vi "Sub_VI_ejecutar_Aula_3.vi"(0 "Serrvicio":u8, 1 "Edif_string_aula":string, 2 "+                 -":bool, 3 "Aula":string, 4 "edo_actual_aula":bool) -> ()   [LabVIEW 2017]
uses:
  GlobalFag.vi
  Global_comSerie.vi
  <vilib>/Instr/_visa.llb/VISA Configure Serial Port (Instr).vi
panel:
  out "aula_ascii":string
  out "estado 3":bool[](array[boolean])
  in  "stop_aula":bool
  in  "Servicios":bool[](array[boolean])
  # "Conf para Edif A, aula 15"
  # "Servicio"
  # "Luz"
  # "+/- Edo. Actual"
  # "Aire"
  # "Proyector"
  # "Agua"
  # "Acceso"
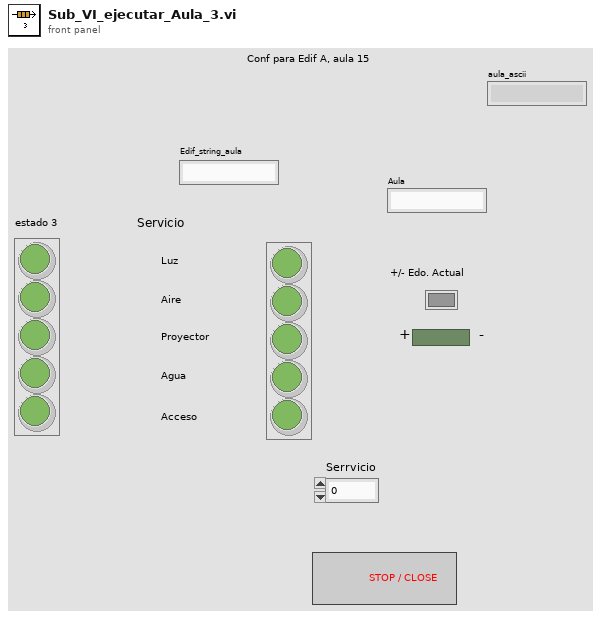
[diagram p1: front panel]
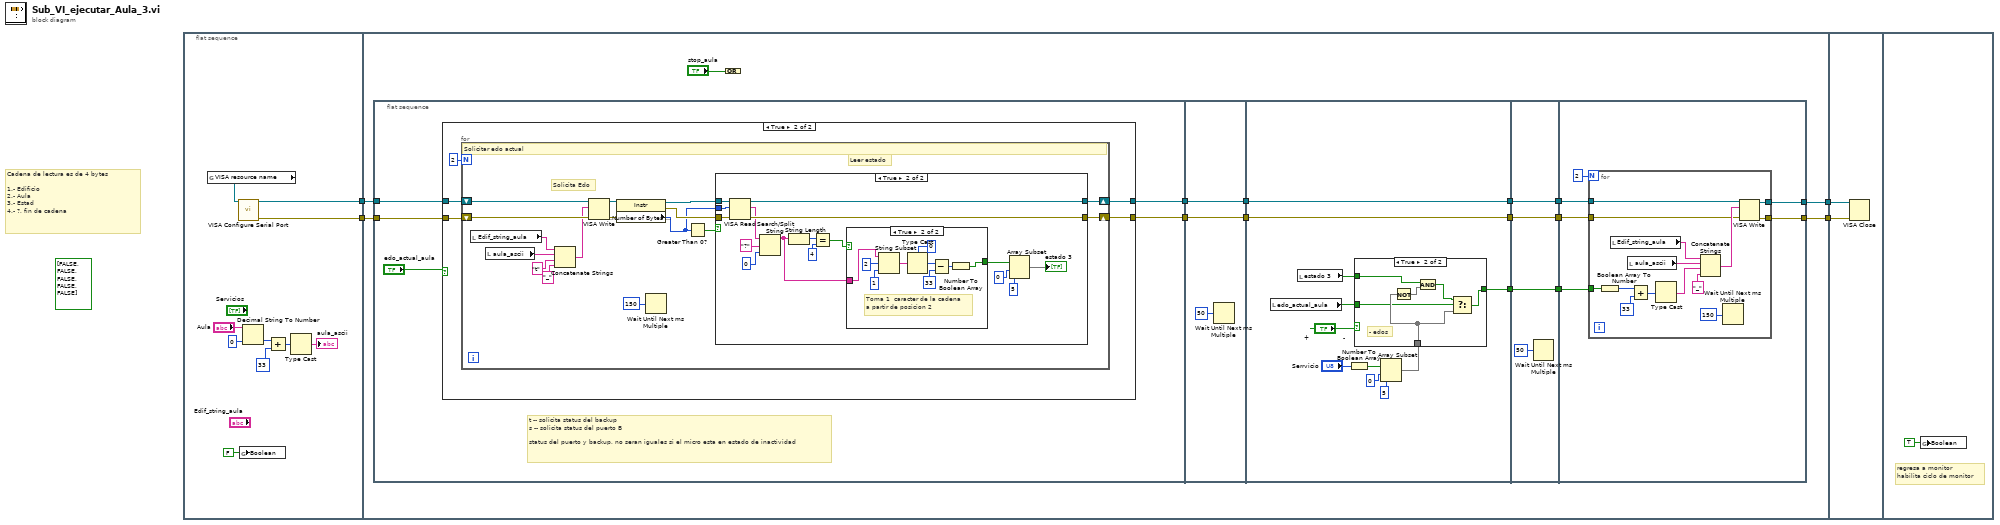
[diagram p0: block diagram]
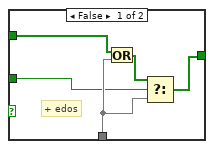
[diagram p5: hidden frame]
diagram:
  (unwired) bool[] [FALSE, FALSE, FALSE, FALSE, FALSE] ("Servicios")
  # "Cadena de lectura es de 4 bytes\n\n1.- Edificio\n2.- Aula\n3.- Estad\n4.- ?, fin de cadena"
  n1 = flat-sequence {
    tunnel: [w14] -> w4
    tunnel: [w13] -> w3
    tunnel: w4 -> [w28]
    tunnel: w3 -> [w27]
    tunnel: [w26] -> w2
    tunnel: [w25] -> w1
    tunnel: w2 -> [w135]
    tunnel: w1 -> [w134]
    frame #0 {
      n2 = global read "Global_comSerie.vi" "VISA resource name"() -> (w11:refnum<visa-resource-name>)
      n3 = call-poly "VISA Configure Serial Port"("VISA resource name"=w11) -> ("VISA resource name out"=w14:refnum<visa-resource-name>, "error out"=w13:errorcluster)  [unwired: 13 in]
      n4 = global write "GlobalFag.vi" "Boolean"(FALSE ("Boolean")) -> ()
      n5 = Decimal String To Number(string="Aula", default (0L)=u8 0 ("default (0 I32)")) -> (number=w8:u8)  [unwired: 1 in, 1 out]
      n6 = Add(x=w8, y=u8 33) -> (x+y=w6:u8)
      n7 = Type Cast(x=w6) -> (*(type *) &x=→"aula_ascii":string)  [unwired: 1 in]
    }
    frame #1 {
      n8 = flat-sequence {
        tunnel: w28 -> [w34]
        tunnel: w27 -> [w33]
        tunnel: [w32] -> w24
        tunnel: [w31] -> w22
        tunnel: w24 -> [w87]
        tunnel: [w87] -> w23
        tunnel: w22 -> [w86]
        tunnel: [w86] -> w21
        tunnel: w23 -> [w95]
        tunnel: w21 -> [w96]
        tunnel: [w97] -> w20
        tunnel: [w96] -> w18
        tunnel: [w95] -> w16
        tunnel: w20 -> [w113]
        tunnel: [w113] -> w19
        tunnel: w18 -> [w112]
        tunnel: [w112] -> w17
        tunnel: w16 -> [w111]
        tunnel: [w111] -> w15
        tunnel: [w119] -> w25
        tunnel: [w118] -> w26
        tunnel: w19 -> [w117]
        tunnel: w17 -> [w115]
        tunnel: w15 -> [w114]
        frame #0 {
          # "t -- solicita status del backup\ns -- solicita status del puerto B\n\nstatus del puerto y backup, no seran iguales si el micro esta en estado de inactividad"
          n9 = case shown="True" "edo_actual_aula" {
            tunnel: w34 -> [w36 w40]
            tunnel: w33 -> [w35 w39]
            tunnel: [w36 w38] -> w32
            tunnel: [w35 w37] -> w31
            frame False {
            }
            frame True {
              n10 = for {
                N: 2 -> [_]
                shift-right: [w55] -> w38
                shift-left: w40 -> [w53]
                shift-right: [w54] -> w37
                shift-left: w39 -> [w52]
                # "Solicita Edo"
                # "Leer estado"
                # "Solicitar edo actual"
                n11 = local read "Edif_string_aula"() -> (w44:string)
                n12 = local read "aula_ascii"() -> (w42:string)
                n13 = Concatenate Strings(w44, w42, "t" ("string"), "_" ("string")) -> (w51:string)
                n14 = VISA Write(VISA resource name=w53, write buffer=w51, error in (no error)=w52) -> (VISA resource name out=w56:refnum<visa-resource-name>, error out=w57:errorcluster)  [unwired: 1 out]
                n15 = property class="Instr"(reference=w56, error in=w57) -> (reference out=w47:refnum<visa-resource-name>, error out=w46:errorcluster, "Serial Settings:Number of Bytes at Serial Port"=w45:u32)
                n16 = Wait Until Next ms Multiple(millisecond multiple=u32 150) -> ()  [unwired: 1 out]
                n17 = Greater Than 0?(x=w45) -> (x > 0?=w48:bool)
                n18 = case shown="True" w48 {
                  tunnel: w47 -> [w58 w75]
                  tunnel: w46 -> [w59 w74]
                  tunnel: [w59 w73] -> w54
                  tunnel: [w58 w72] -> w55
                  tunnel: w45 -> [_ w71]
                  frame False {
                  }
                  frame True {
                    n19 = VISA Read(VISA resource name=w75, byte count=w71, error in (no error)=w74) -> (VISA resource name out=w72:refnum<visa-resource-name>, read buffer=w67:string, error out=w73:errorcluster)  [unwired: 1 out]
                    n20 = Search/Split String(string=w67, search string/char (-)="?", offset (0)=u8 0) -> (substring before match=w64:string)  [unwired: 2 out]
                    n21 = String Length(string=w64) -> (length=w70:i32)
                    n22 = Equal?(x=w70, y=4) -> (x = y?=w65:bool)
                    n23 = case shown="True" w65 {
                      tunnel: [_ w77] -> w61
                      tunnel: w64 -> [_ w76]
                      frame False {
                      }
                      frame True {
                        # "Toma 1  caracter de la cadena\na partir de posicion 2"
                        n24 = String Subset(string=w76, offset (0)=2, length (rest)=1 ("length (rest)")) -> (substring=w81:string)
                        n25 = Type Cast(type=u8 0 ("width (-)"), x=w81) -> (*(type *) &x=w79:u8)
                        n26 = Subtract(x=w79, y=u8 33) -> (x-y=w80:u8)
                        n27 = Number To Boolean Array(number=w80) -> (Boolean array=w77:bool[])
                      }
                    }
                    n28 = Array Subset(array=w61, index=0, length=5) -> (→"estado 3":bool[])
                  }
                }
              }
            }
          }
        }
        frame #1 {
          n29 = Wait Until Next ms Multiple(millisecond multiple=u32 50) -> ()  [unwired: 1 out]
        }
        frame #2 {
          n30 = local read "edo_actual_aula"() -> (w93:bool)
          n31 = local read "estado 3"() -> (w92:bool[])
          n32 = Number To Boolean Array(number="Serrvicio") -> (Boolean array=w89:bool[])
          n33 = Array Subset(array=w89, index=0, length=5) -> (w88:bool[])
          n34 = case shown="True" "+                 -" {
            tunnel: w88 -> [w101 w107]
            tunnel: [w103 w105] -> w97
            tunnel: w93 -> [w100 w106]
            tunnel: w92 -> [w99 w104]
            frame False {
              # "+ edos"
              n35 = Or(x=w99, y=w101) -> (x .or. y?=w102:bool[])
              n36 = Select(t=w102, s=w100, f=w101) -> (s? t:f=w103:bool[])
            }
            frame True {
              # "- edos"
              n37 = Not(x=w107) -> (.not. x?=w109:bool[])
              n38 = And(x=w104, y=w109) -> (x .and. y?=w108:bool[])
              n39 = Select(t=w108, s=w106, f=w107) -> (s? t:f=w105:bool[])
            }
          }
        }
        frame #3 {
          n40 = Wait Until Next ms Multiple(millisecond multiple=u32 50) -> ()  [unwired: 1 out]
        }
        frame #4 {
          n41 = for {
            N: 2 -> [_]
            tunnel: [w133] -> w119
            tunnel: [w132] -> w118
            tunnel: w117 -> [w125]
            tunnel: w115 -> [w124]
            tunnel: w114 -> [w123]
            n42 = Boolean Array To Number(Boolean array=w125) -> (number=w126:u8)
            n43 = local read "Edif_string_aula"() -> (w122:string)
            n44 = local read "aula_ascii"() -> (w121:string)
            n45 = Add(x=w126, y=u8 33) -> (x+y=w129:u8)
            n46 = Type Cast(x=w129) -> (*(type *) &x=w128:string)  [unwired: 1 in]
            n47 = Concatenate Strings(w122, w121, w128, "_" ("string")) -> (w131:string)
            n48 = Wait Until Next ms Multiple(millisecond multiple=u32 150) -> ()  [unwired: 1 out]
            n49 = VISA Write(VISA resource name=w123, write buffer=w131, error in (no error)=w124) -> (VISA resource name out=w132:refnum<visa-resource-name>, error out=w133:errorcluster)  [unwired: 1 out]
          }
        }
      }
      n50 = Compound Arithmetic op=OR("stop_aula") -> ()  [unwired: 1 out]
    }
    frame #2 {
      n51 = VISA Close(VISA resource name=w135, error in (no error)=w134) -> ()  [unwired: 1 out]
    }
    frame #3 {
      # "regresa a monitor\nhabilita ciclo de monitor"
      n52 = global write "GlobalFag.vi" "Boolean"(TRUE ("Boolean")) -> ()
    }
  }
